vi "Gather Input.vi"(4 "Shifter":T1, 6 "Gamepad":T1, 8 "Joystick Right":T1, 11 "Joystick Left":T1) -> ()   [LabVIEW 2017]
uses:
  <vilib>/Rock Robotics/WPI/Joystick/WPI_JoystickDevRef.ctl
  <vilib>/Rock Robotics/WPI/Joystick/WPI_JoystickDeviceEnum.ctl
  Joystick Values.vi
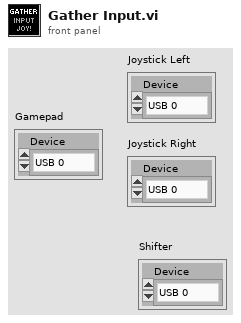
[diagram p1: front panel]
types:
  T1 = typedef "WPI_JoystickDevRef.ctl" = cluster{"Device":T2}
  T2 = typedef "WPI_JoystickDeviceEnum.ctl" = enum16{"USB 0", "USB 1", "USB 2", "USB 3", "USB 4", "USB 5"}
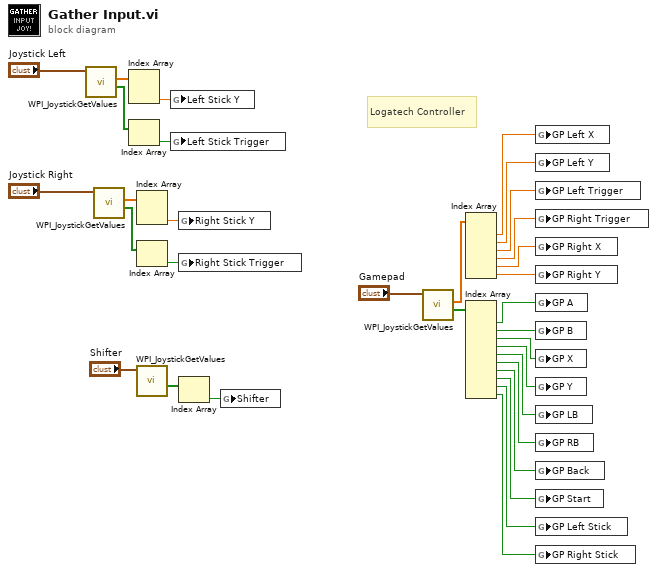
[diagram p0: block diagram]
diagram:
  # "Logatech Controller"
  n1 = call <vilib>:"WPI_JoystickGetValues.vi"("JoystickDevRef"="Joystick Left") -> ("Buttons"=w24:bool[], "Axes"=w23:dbl[])  [unwired: 6 in, 3 out]
  n2 = call <vilib>:"WPI_JoystickGetValues.vi"("JoystickDevRef"="Joystick Right") -> ("Buttons"=w30:bool[], "Axes"=w28:dbl[])  [unwired: 6 in, 3 out]
  n3 = Index Array(array=w23) -> (element #2=w25:dbl)  [unwired: 2 in, 1 out]
  n4 = Index Array(array=w24) -> (element=w26:bool)  [unwired: 1 in]
  n5 = Index Array(array=w28) -> (element #2=w27:dbl)  [unwired: 2 in, 1 out]
  n6 = Index Array(array=w30) -> (element=w29:bool)  [unwired: 1 in]
  n7 = call <vilib>:"WPI_JoystickGetValues.vi"("JoystickDevRef"="Shifter") -> ("Buttons"=w21:bool[])  [unwired: 6 in, 4 out]
  n8 = global write "Joystick Values.vi" "Left Stick Y"(w25) -> ()
  n9 = global write "Joystick Values.vi" "Left Stick Trigger"(w26) -> ()
  n10 = global write "Joystick Values.vi" "Right Stick Y"(w27) -> ()
  n11 = global write "Joystick Values.vi" "Right Stick Trigger"(w29) -> ()
  n12 = Index Array(array=w21) -> (element=w20:bool)  [unwired: 1 in]
  n13 = global write "Joystick Values.vi" "Shifter"(w20) -> ()
  n14 = call <vilib>:"WPI_JoystickGetValues.vi"("JoystickDevRef"="Gamepad") -> ("Buttons"=w18:bool[], "Axes"=w6:dbl[])  [unwired: 6 in, 3 out]
  n15 = Index Array(array=w6) -> (element #1=w7:dbl, element #2=w5:dbl, element #3=w2:dbl, element #4=w1:dbl, element #5=w4:dbl, element #6=w3:dbl)  [unwired: 6 in]
  n16 = Index Array(array=w18) -> (element #1=w17:bool, element #2=w16:bool, element #3=w15:bool, element #4=w14:bool, element #5=w13:bool, element #6=w12:bool, element #7=w11:bool, element #8=w10:bool, element #9=w9:bool, element #10=w8:bool)  [unwired: 10 in]
  n17 = global write "Joystick Values.vi" "GP Left X"(w7) -> ()
  n18 = global write "Joystick Values.vi" "GP Left Y"(w5) -> ()
  n19 = global write "Joystick Values.vi" "GP Left Trigger"(w2) -> ()
  n20 = global write "Joystick Values.vi" "GP Right Trigger"(w1) -> ()
  n21 = global write "Joystick Values.vi" "GP Right X"(w4) -> ()
  n22 = global write "Joystick Values.vi" "GP Right Y"(w3) -> ()
  n23 = global write "Joystick Values.vi" "GP A"(w17) -> ()
  n24 = global write "Joystick Values.vi" "GP B"(w16) -> ()
  n25 = global write "Joystick Values.vi" "GP X"(w15) -> ()
  n26 = global write "Joystick Values.vi" "GP Y"(w14) -> ()
  n27 = global write "Joystick Values.vi" "GP LB"(w13) -> ()
  n28 = global write "Joystick Values.vi" "GP RB"(w12) -> ()
  n29 = global write "Joystick Values.vi" "GP Back"(w11) -> ()
  n30 = global write "Joystick Values.vi" "GP Start"(w10) -> ()
  n31 = global write "Joystick Values.vi" "GP Left Stick"(w9) -> ()
  n32 = global write "Joystick Values.vi" "GP Right Stick"(w8) -> ()
